vi "Kepco cfg current.vi"(8 "error in (no error)":errorcluster {"code" format="%.0x"}, 9 "Simulation":T1, 10 "Channel parsed command info":T2, 11 "input cluster":refnum<class "KepcoBOP.lvclass">) -> (0 "error out":errorcluster, 2 "new commands":string, 3 "output cluster":refnum<class "KepcoBOP.lvclass">)   [LabVIEW 2020, in "KepcoBOP.lvclass"]
uses:
  KepcoBOP.lvclass
  Shared/Device Driver/channel parsed cmd cluster.ctl
  shared/OnOffTypeDef.ctl
  KepcoBOP.lvclass/KepcoBOP.ctl
  shared/CompressAndUpdate(Poly)/CompressAndUpdate(Numeric).vi
panel:
  out "Numeric":i32
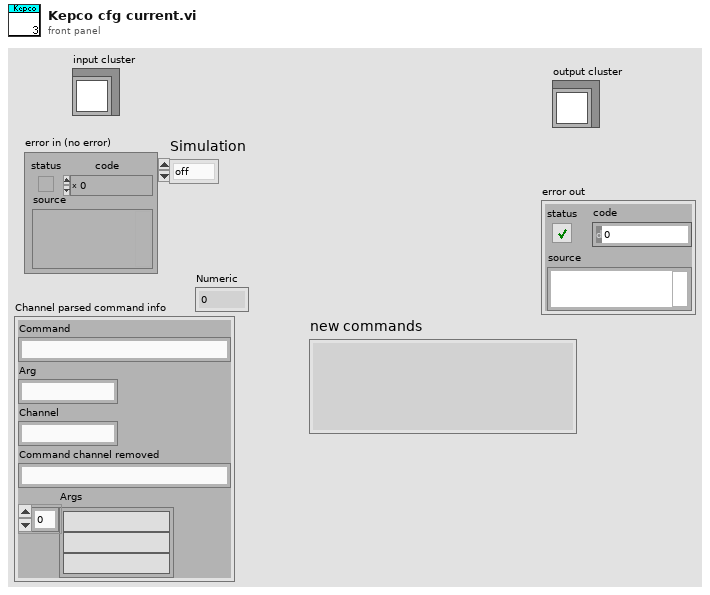
[diagram p1: front panel]
types:
  T1 = typedef "OnOffTypeDef.ctl" = enum16{"off", "on"}
  T2 = typedef "channel parsed cmd cluster.ctl" = cluster{"Command":string, "Arg":string, "Channel":string, "Command channel removed":string, "Args":string[]}
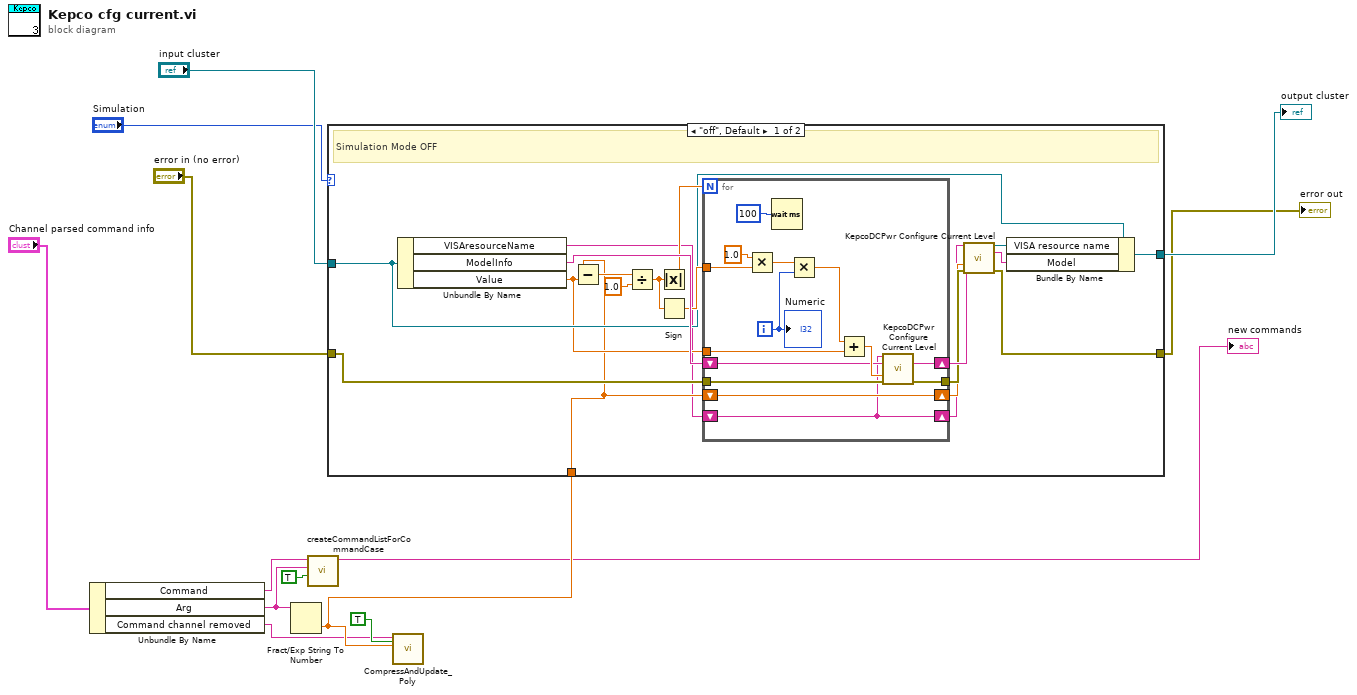
[diagram p0: block diagram]
diagram:
  n1 = Unbundle By Name("Channel parsed command info") -> ("Command"=w11:string, "Arg"=w13:string, "Command channel removed"=w1:string)
  n2 = Fract/Exp String To Number(string=w13) -> (number=w9:dbl)  [unwired: 3 in, 1 out]
  n3 = call "createCommandListForCommandCase.vi"("immediate Check (only once)"=TRUE, "setvalue"=w13, "command"=w11) -> ("new commands"=→"new commands":string)  [unwired: 8 in]
  n4 = case shown="\"off\", Default" "Simulation" {
    tunnel: [w16 w47] -> w5
    tunnel: w9 -> [w18 _]
    tunnel: "input cluster" -> [w22 w48]
    tunnel: "error in (no error)" -> [w19 w47]
    tunnel: [w21 w48] -> w6
    frame "off", Default {
      # "Simulation Mode OFF"
      n5 = Unbundle By Name(w22) -> ("VISAresourceName"=w15:string, "ModelInfo"=w32:string, "Value"=w20:dbl)
      n6 = Subtract(x=w18, y=w20) -> (x-y=w27:dbl)
      n7 = Divide(x=w27, y=1.0) -> (x/y=w24:dbl)
      n8 = Absolute Value(x=w24) -> (abs(x)=w23:dbl)
      n9 = Sign(1:w24) -> (0:w25:dbl)
      n10 = for {
        N: w23 -> [_]
        tunnel: w25 -> [w45]
        tunnel: [w42] -> w30
        tunnel: w20 -> [w37]
        tunnel: w19 -> [w35]
        shift-right: [w34] -> w17
        shift-left: w18 -> [w34]
        shift-right: [w33] -> w14
        shift-left: w15 -> [w33]
        shift-right: [w46] -> w31
        shift-left: w32 -> [w36]
        i -> [w39]
        n11 = Multiply(x=1.0 ("y"), y=w45) -> (x*y=w40:dbl)
        n12 = Wait (ms)(milliseconds to wait=u32 100) -> ()  [unwired: 1 out]
        n13 = Multiply(x=w40, y=w39) -> (x*y=w38:dbl)
        n14 = Add(x=w38, y=w37) -> (x+y=w43:dbl)
        n15 = call "KepcoDCPwr Configure Current Level.vi"("VISA Session"=w33, "Model In"=w36, "level (0.0 volts)"=w43, "error in (no error)"=w35) -> ("Model Out"=w46:string, "error out"=w42:errorcluster)  [unwired: 8 in, 2 out]
        "Numeric" <- w39
      }
      n16 = call "KepcoDCPwr Configure Current Level.vi"("VISA Session"=w14, "Model In"=w31, "level (0.0 volts)"=w17, "error in (no error)"=w30) -> ("VISA Session Out"=w28:refnum<visa-resource-name>, "Model Out"=w29:string, "error out"=w16:errorcluster)  [unwired: 8 in, 1 out]
      n17 = Bundle By Name(cluster=w22, "VISA resource name"=w28, "Model"=w29) -> (w21:refnum<class "KepcoBOP.lvclass">)
    }
    frame "on" {
      # "Simulation Mode ON"
    }
  }
  "output cluster" <- w6
  "error out" <- w5
  n18 = call-poly "CompressAndUpdate_Poly.vi"("force CVT update (false)"=TRUE ("force CVT update"), "Numeric"=w9, "command or variable name"=w1) -> ()  [unwired: 8 in, 1 out]
